vi "19572_get_test_times.vi"(8 "error in (no error)":errorcluster, 9 "modes":string[](array[string]), 10 "steps":u16[](array[numeric]), 11 "VISA Refnum in":refnum<visa-resource-name>) -> (0 "error out":errorcluster, 2 "times":string[](array[string]), 3 "VISA Refnum out":refnum<visa-resource-name>)   [LabVIEW 2015]
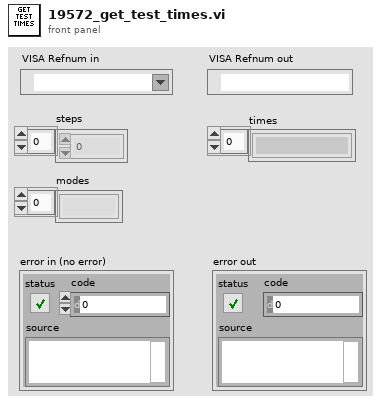
[diagram p1: front panel]
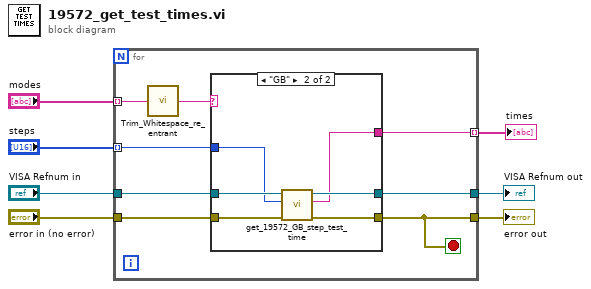
[diagram p0: block diagram]
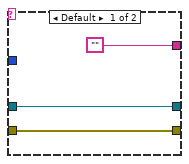
[diagram p2: hidden frame]
diagram:
  n1 = for {
    tunnel: "steps" -> [w15] mode=indexing
    tunnel: "VISA Refnum in" -> [w14]
    tunnel: "error in (no error)" -> [w13]
    tunnel: [w10] -> w5
    tunnel: [w12] -> w6 mode=indexing
    tunnel: [w9] -> w7
    tunnel: "modes" -> [w8] mode=indexing
    stop <- w10 stop-if-true
    n2 = call "Trim_Whitespace_re_entrant.vi"("string"=w8) -> ("trimmed string"=w11:string)  [unwired: 3 in]
    n3 = case shown="\"GB\"" w11 {
      tunnel: w15 -> [_ w22]
      tunnel: w14 -> [w16 w24]
      tunnel: w13 -> [w18 w20]
      tunnel: [w18 w19] -> w10
      tunnel: ["" w21] -> w12
      tunnel: [w16 w23] -> w9
      frame Default {
      }
      frame "GB" {
        n4 = call "get_19572_GB_step_test_time.vi"("error in (no error)"=w20, "step"=w22, "VISA resource in"=w24) -> ("error out"=w19:errorcluster, "GB total time"=w21:string, "VISA resource out"=w23:refnum<visa-resource-name>)  [unwired: 6 in]
      }
    }
  }
  "VISA Refnum out" <- w7
  "times" <- w6
  "error out" <- w5
